vi "Read.vi"() -> ()   [LabVIEW 2018]
uses:
  <vilib>/Utility/file.llb/Read Delimited Spreadsheet (string).vi
panel:
  out "all rows":string[][](array[string]) caption="모든 행"
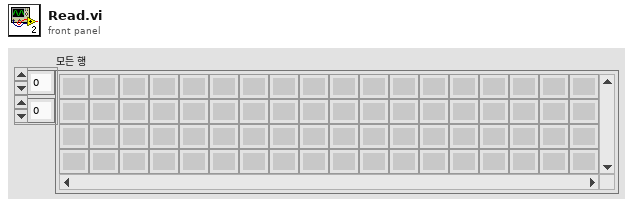
[diagram p1: front panel]
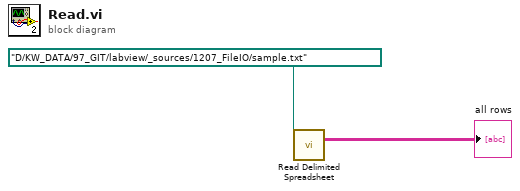
[diagram p0: block diagram]
diagram:
  n1 = call-poly <vilib>:"Read Delimited Spreadsheet.vi"("file path (dialog if empty)"=path "D:/KW_DATA/97_GIT/labview/_sources/1207_FileIO/sample.txt") -> ("all rows"=→"all rows":string[][])  [unwired: 9 in, 5 out]
